vi "Test Tokenizer Relative Formats.vi"(8 "error in (no error)":errorcluster) -> (0 "error out":errorcluster)   [LabVIEW 2019]
uses:
  <vilib>/addons/_JKI Toolkits/Caraya/classes/Test/Test.lvclass
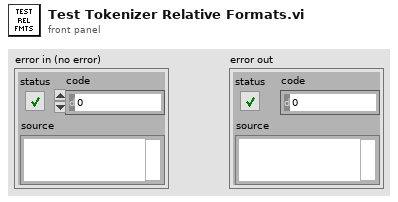
[diagram p1: front panel]
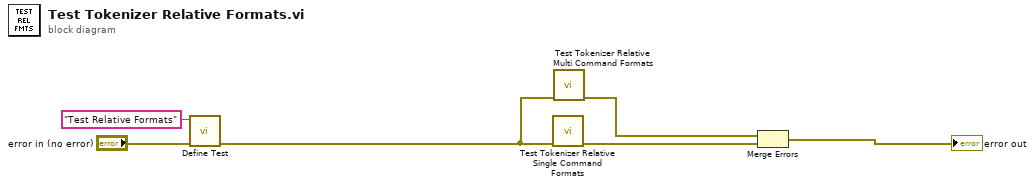
[diagram p0: block diagram]
diagram:
  n1 = call <vilib>:"Define Test.vi"("error in (no error)"="error in (no error)", "Label (VI Title)"="Test Relative Formats") -> ("error out"=w3:errorcluster)  [unwired: 8 in, 1 out]
  n2 = call "Test Tokenizer Relative Single Command Formats.vi"("error in (no error)"=w3) -> ("error out"=w5:errorcluster)  [unwired: 10 in]
  n3 = call "Test Tokenizer Relative Multi Command Formats.vi"("error in (no error)"=w3) -> ("error out"=w1:errorcluster)  [unwired: 10 in]
  n4 = Merge Errors(w1, w5) -> (→"error out":errorcluster)
